vi "Queue Monitor.vi"   [LabVIEW 2023]
doc: "This VI looks at all the open queue references and collects their statuses."
uses:
  <vilib>/Platform/TimedLoop/XDataNode/timing_clust.ctl
  <vilib>/Platform/TimedLoop/XDataNode/nitl_modes.ctl
  <vilib>/Platform/TimedLoop/XDataNode/wakeup.ctl
  Type Definitions/Payload Class.ctl
  Type Definitions/Enumerated Constants/Software Monitor.ctl
  Type Definitions/Queue Monitor.ctl
  <vilib>/platform/TimedLoop/XDataNode/XDataNode.xnode
  <vilib>/Platform/TimedLoop/XDataNode/XDNodeRunTimeDep.lvlib
types:
  T1 = typedef "XDNodeRunTimeDep.lvlib/timing_clust.ctl" = cluster{"Expected End [f-1]":u64, "Actual End [f-1]":u64, "Finished Late? [f-1]":bool, "Expected End [i-1]":u64, "Actual End [i-1]":u64, "Finished Late? [i-1]":bool, "Expected Start [i]":u64, "Actual Start [i]":u64, "Expected Start [f]":u64, "Actual Start [f]":u64, "Source Name":string, "Structure Name":string, "Period":i64, "Deadline":i64, "Offset":i64, "Start":i64, "Priority":i32, "Timeout":i32, "Mode":T2, "Wakeup Reason":T3, "Error":errorcluster, "Source Type":string, "Secondary Source Type":string, "Global End Time":u64, "Global Start Time":u64, "Frame Duration":u64, "Iteration Duration":u64, "Assigned CPU":i32, "I/O Scan Engine Mode":u32}
  T2 = typedef "XDNodeRunTimeDep.lvlib/nitl_modes.ctl" = enum32{"No Change", "Process missed periods, maintain original phase", "Discard missed periods, maintain original phase", "Process missed periods, ignore original phase", "Discard missed periods, ignore original phase"}
  T3 = typedef "XDNodeRunTimeDep.lvlib/wakeup.ctl" = enum32{"Normal", "Aborted", "Asynchronous wakeup", "Timing source error", "Timed loop error", "Timeout"}
  T4 = typedef "Software Monitor.ctl" = enum16{"Internet Connection Monitor", "CPU Monitor", "Archive Monitor", "Memory Monitor", "Queue Monitor", "RTOS Update", "RTOS Monitor"}
  T5 = typedef "Payload Class.ctl" = enum16{"System State", "Parameters", "Metadata", "Software Monitor", "Data", "Commands"}
  T6 = typedef "Queue Monitor.ctl" = cluster{"Queue Name":string, "Max Queue Size":i32, "Pending Remove":i32, "Pending Insert":i32, "Elements in Queue":i32}
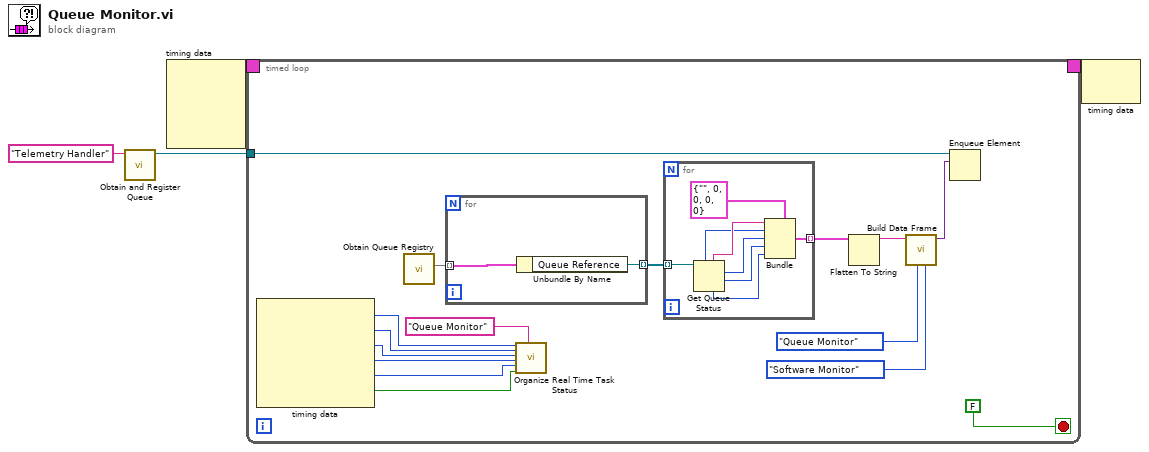
[diagram p0: block diagram]
diagram:
  n1 = call "Obtain and Register Queue.vi"("Queue Name (unnamed)"="Telemetry Handler" ("name (unnamed)")) -> ("Queue Reference"=w2:refnum<queue>)  [unwired: 9 in, 1 out]
  n2 = node-c288() -> (w4:T1)  [unwired: 4 in]
  n3 = timed-loop {
    timing: w4 -> [_]
    timing-out: [_] -> w3
    tunnel: w2 -> [w15]
    stop <- FALSE stop-if-true
    n4 = node-c288() -> (w12:i32, w11:i32, w10:i64, w9:i64, w8:i64, w7:bool)  [unwired: 1 in]
    n5 = call "Obtain Queue Registry.vi"() -> ("Queue Registry"=w6:map{string, refnum<queue>})  [unwired: 9 in, 2 out]
    n6 = for {
      tunnel: w6 -> [w22] mode=indexing
      tunnel: [w21] -> w5 mode=indexing
      n7 = Unbundle By Name(w22) -> ("Queue Reference"=w21:refnum<queue>)
    }
    n8 = call "Organize Real Time Task Status.vi"("Priority"=w12, "Processor"=w11, "Offset"=w10, "Iteration Duration"=w9, "Period"=w8, "Finished Late? [i-1]"=w7, "Task Name"="Queue Monitor") -> ()  [unwired: 12 in, 1 out]
    n9 = for {
      tunnel: w5 -> [w37] mode=indexing
      tunnel: [w31] -> w16 mode=indexing
      n10 = Get Queue Status(queue=w37) -> (queue name=w36:string, max queue size=w35:i32, # pending remove=w34:i32, # pending insert=w33:i32, # elements in queue=w32:i32)  [unwired: 2 in, 3 out]
      n11 = Bundle(cluster=T6 {"Queue Name"="", "Max Queue Size"=0, "Pending Remove"=0, "Pending Insert"=0, "Elements in Queue"=0}, "Queue Name"=w36, "Max Queue Size"=w35, "Pending Remove"=w34, "Pending Insert"=w33, "Elements in Queue"=w32) -> (w31:T6)
    }
    n12 = Flatten To String(anything=w16) -> (data string=w19:string)  [unwired: 3 in, 2 out]
    n13 = call "Build Data Frame.vi"("Payload Class (Data)"=Payload_Class."Software Monitor", "Payload ID (0)"=Software_Monitor."Queue Monitor", "Payload (Empty String)"=w19) -> ("Frame"=w14:variant)  [unwired: 7 in, 1 out]
    n14 = Enqueue Element(queue=w15, element=w14) -> ()  [unwired: 2 in, 3 out]
  }
  n15 = node-c288(w3) -> ()  [unwired: 1 out]
